vi "Create temporary file name.vi"(6 "Temporary Image File":T1=enum.".jpeg", 7 "Flush Files (F)":bool, 8 "error in (no error)":errorcluster, 9 "msec (F)":bool, 10 "hh:mm:ss (false)":bool, 11 "Dir path":path) -> (0 "error out":errorcluster, 3 "File path":path)   [LabVIEW 2020, in "Exaprom PDF.lvlib"]
doc: "Version 1.0\nDeveloped by Jean-Marc Simard\nCopyright © 2010, Exaprom Inc.\nAll rights reserved.\nLicense: BSD"
uses:
  <userlib>/labview-PDF-writer-master/Exaprom PDF.lvlib
  <userlib>/labview-PDF-writer-master/Controls/File Path Controls/Temporary File.ctl
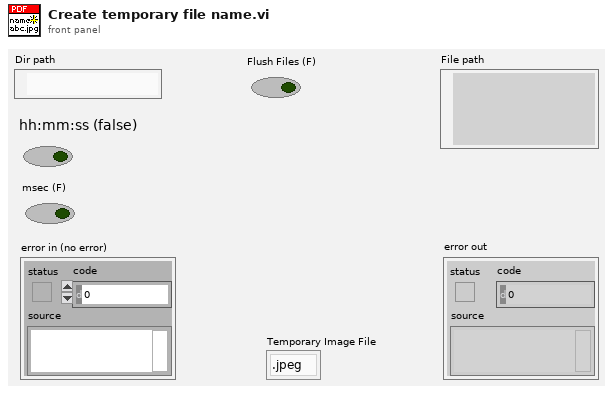
[diagram p1: front panel]
types:
  T1 = typedef "Exaprom PDF.lvlib/Temporary File.ctl" = enum16{".bmp", ".jpeg", ".png", ".pdf", "No File", ".xml"}
  T2 = typedef "LVDateTimeRec.ctl" = cluster{"fractional second":dbl, "second":i32, "minute":i32, "hour":i32, "day of month":i32, "month":i32, "year":i32, "day of week":i32, "day of year":i32, "DST":i32}
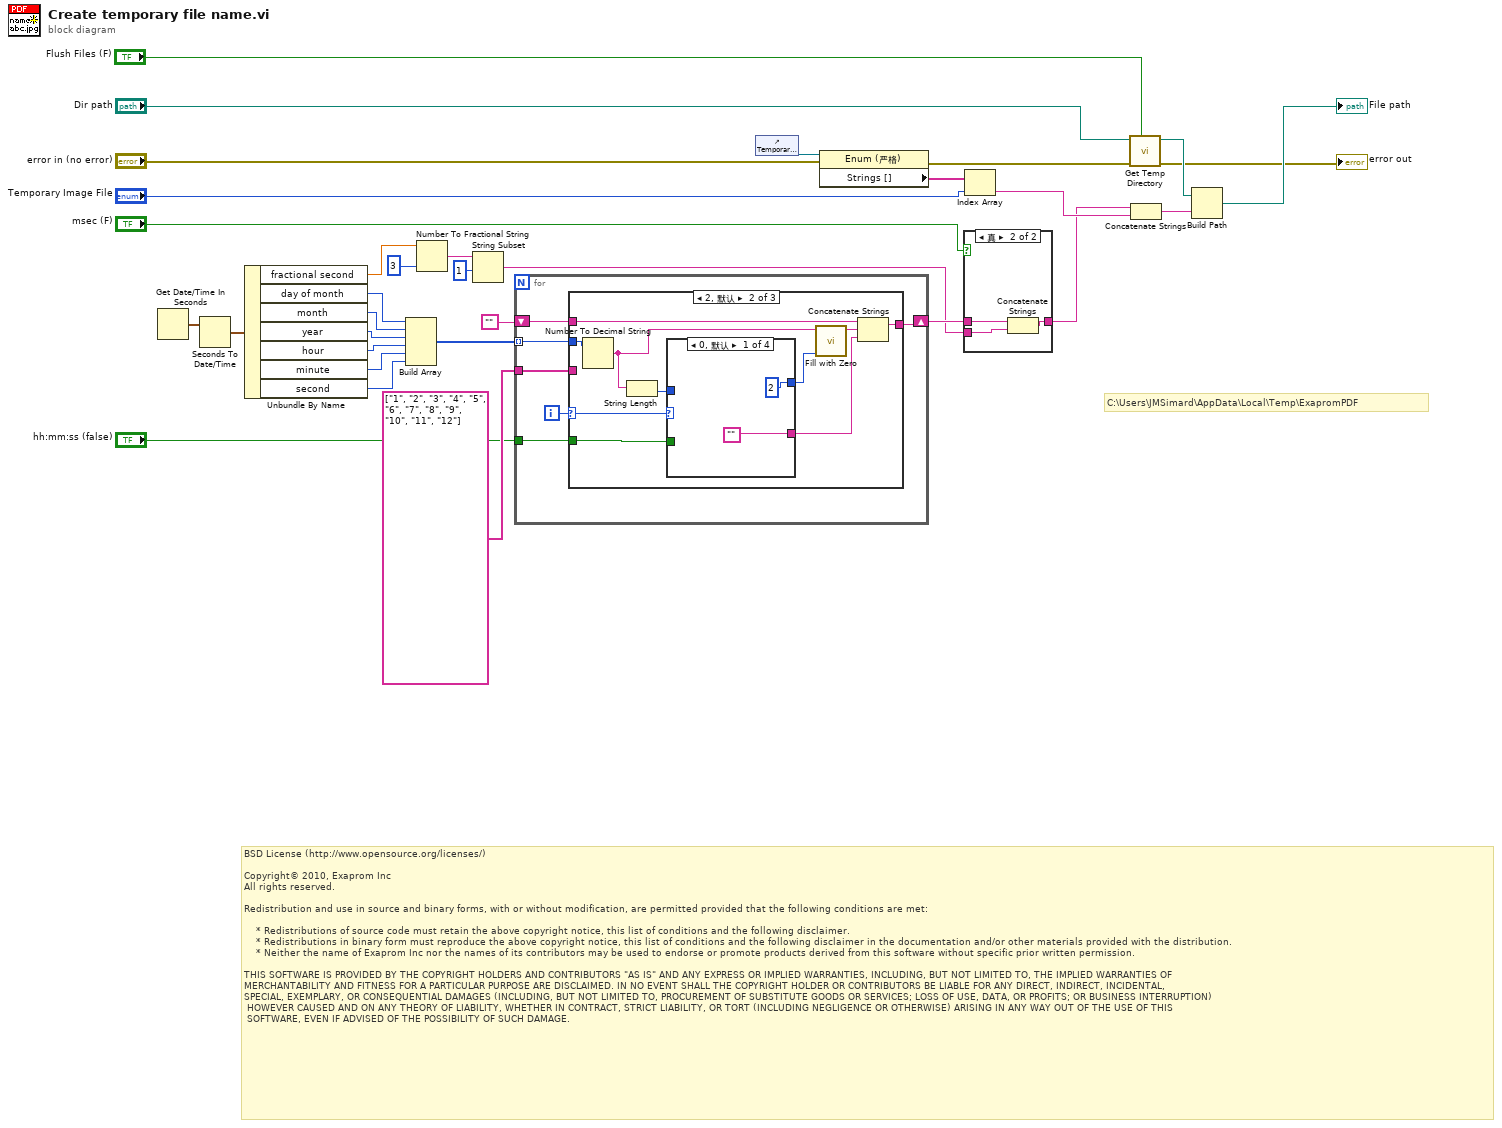
[diagram p0: block diagram]
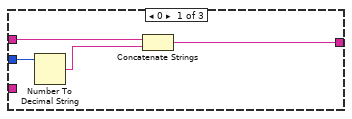
[diagram p3: hidden frame]
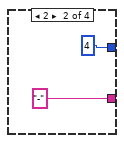
[diagram p4: hidden frame]
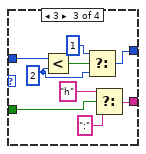
[diagram p5: hidden frame]
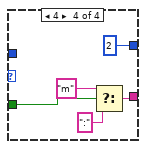
[diagram p6: hidden frame]
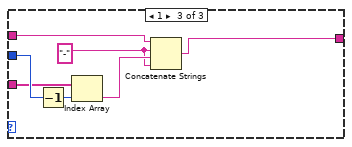
[diagram p7: hidden frame]
diagram:
  # "C:\\Users\\JMSimard\\AppData\\Local\\Temp\\ExapromPDF"
  # "BSD License (http://www.opensource.org/licenses/)\n\nCopyright© 2010, Exaprom Inc\nAll rights reserved.\n\nRedistribution and use in source and binary forms, with or without modification, are permitted provided that the following conditions are met:\n\n    * Redistributions of source code must retain the above copyright notice, this list of conditions and the following disclaimer.\n    * Redistributions in binary form must reproduce the above copyright notice, this list of conditions and the following disclaimer in the documentation and/or other materials provided with the distribution.\n    * Neither the name of Exaprom Inc nor the names of its contributors may be used to endorse or promote products derived from this software without specific prior written permission.\n\nTHIS SOFTWARE IS PROVIDED BY THE COPYRIGHT HOLDERS AND CONTRIBUTORS \"AS IS\" AND ANY EXPRESS OR IMPLIED WARRANTIES, INCLUDING, BUT NOT LIMITED TO, THE IMPLIED WARRANTIES OF \nMERCHANTABILITY AND FITNESS FOR A PARTICULAR PURPOSE ARE DISCLAIMED. IN NO EVENT SHALL THE COPYRIGHT HOLDER OR CONTRIBUTORS BE LIABLE FOR ANY DIRECT, INDIRECT, INCIDENTAL,\nSPECIAL, EXEMPLARY, OR CONSEQUENTIAL DAMAGES (INCLUDING, BUT NOT LIMITED TO, PROCUREMENT OF SUBSTITUTE GOODS OR SERVICES; LOSS OF USE, DATA, OR PROFITS; OR BUSINESS INTERRUPTION)\n HOWEVER CAUSED AND ON ANY THEORY OF LIABILITY, WHETHER IN CONTRACT, STRICT LIABILITY, OR TORT (INCLUDING NEGLIGENCE OR OTHERWISE) ARISING IN ANY WAY OUT OF THE USE OF THIS\n SOFTWARE, EVEN IF ADVISED OF THE POSSIBILITY OF SUCH DAMAGE."
  n1 = Get Date/Time In Seconds() -> (seconds since 1Jan1904=w32:timestamp)
  n2 = Seconds To Date/Time(time stamp (now)=w32) -> (date time rec=w31:T2)  [unwired: 1 out]
  n3 = Unbundle By Name(w31) -> ("fractional second"=w20:dbl, "day of month"=w30:i32, "month"=w29:i32, "year"=w28:i32, "hour"=w27:i32, "minute"=w26:i32, "second"=w25:i32)
  n4 = Build Array(w30, w29, w28, w27, w26, w25) -> (w24:i32[])
  n5 = Number To Fractional String(number=w20, precision (6)=i16 3) -> (F-format string=w19:string)  [unwired: 2 out]
  n6 = String Subset(string=w19, offset (0)=1) -> (substring=w15:string)  [unwired: 1 out]
  n7 = for {
    tunnel: w24 -> [w35] mode=indexing
    tunnel: string[] ["1", "2", "3", "4", "5", "6", "7", "8", "9", "10", "11", "12"] -> [w37]
    shift-right: [w34] -> w21
    shift-left: "" -> [w36]
    tunnel: "hh:mm:ss (false)" -> [w33]
    i -> [w38]
    n8 = case shown="2, 默认" w38 {
      selector: w38 -> [_ w49 _]
      tunnel: w37 -> [_ _ w76]
      tunnel: w36 -> [w41 w51 w75]
      tunnel: w35 -> [w42 w52 w77]
      tunnel: [w40 w50 w73] -> w34
      tunnel: w33 -> [_ w47 _]
      frame 0 {
        n9 = Number To Decimal String(number=w42) -> (decimal integer string=w39:string)  [unwired: 1 out]
        n10 = Concatenate Strings(w41, w39) -> (w40:string)
      }
      frame 2, Default {
        n11 = Number To Decimal String(number=w52) -> (decimal integer string=w44:string)  [unwired: 1 out]
        n12 = String Length(string=w44) -> (length=w43:i32)
        n13 = case shown="0, 默认" w49 {
          tunnel: ["" "-" w63 w68] -> w48
          tunnel: w47 -> [_ _ w64 w67]
          tunnel: [2 4 w59 2] -> w45
          tunnel: w43 -> [_ _ w61 _]
          frame 0, Default {
          }
          frame 2 {
          }
          frame 3 {
            w58 = 2 ("y")
            n14 = Less?(x=w61, y=w58) -> (x < y?=w60:bool)
            n15 = Select(t=1, s=w60, f=w58) -> (s? t:f=w59:i32)
            n16 = Select(t="h", s=w64, f=":") -> (s? t:f=w63:string)
          }
          frame 4 {
            n17 = Select(t="m", s=w67, f=":") -> (s? t:f=w68:string)
          }
        }
        n18 = call <userlib>:"Fill with Zero.vi"("Nbre caractères"=w45, "String IN"=w44) -> ("String OUT"=w46:string)  [unwired: 9 out]
        n19 = Concatenate Strings(w51, w46, w48) -> (w50:string)
      }
      frame 1 {
        w71 = "-"
        n20 = Decrement(x=w77) -> (x-1=w72:i32)
        n21 = Index Array(array=w76, index=w72) -> (element=w74:string)
        n22 = Concatenate Strings(w75, w71, w74, w71) -> (w73:string)
      }
    }
  }
  n23 = control-ref of="Temporary Image File"() -> (w11:refnum<vi>)
  n24 = property class="Enum (严格)"(reference=w11, error in="error in (no error)") -> (error out=w7:errorcluster, "Strings []"=w10:string[])  [unwired: 1 out]
  n25 = case shown="真" "msec (F)" {
    tunnel: w21 -> [w78 w81]
    tunnel: [w78 w80] -> w8
    tunnel: w15 -> [_ w79]
    frame False {
    }
    frame True {
      n26 = Concatenate Strings(w81, w79) -> (w80:string)
    }
  }
  n27 = Index Array(array=w10, index="Temporary Image File") -> (element=w9:string)
  n28 = call <userlib>:"Get Temp Directory.vi"("Flush Files (F)"="Flush Files (F)", "error in (no error)"=w7, "Dir path"="Dir path") -> ("error out"=→"error out":errorcluster, "created path"=w12:path)  [unwired: 7 out]
  n29 = Concatenate Strings(w8, w9) -> (w13:string)
  n30 = Build Path(base path=w12, name or relative path=w13) -> (appended path=→"File path":path)
